vi "set origin.vi"(8 "error in (no error)":errorcluster, 11 "StageMG100204SutterMP285 in":refnum<class "StageMG100204SutterMP285.lvclass">=refnum) -> (0 "error out":errorcluster, 3 "StageMG100204SutterMP285 out":refnum<class "StageMG100204SutterMP285.lvclass">)   [LabVIEW 2010, in "StageMG100204SutterMP285.lvclass"]
uses:
  StageMG100204SutterMP285.lvclass
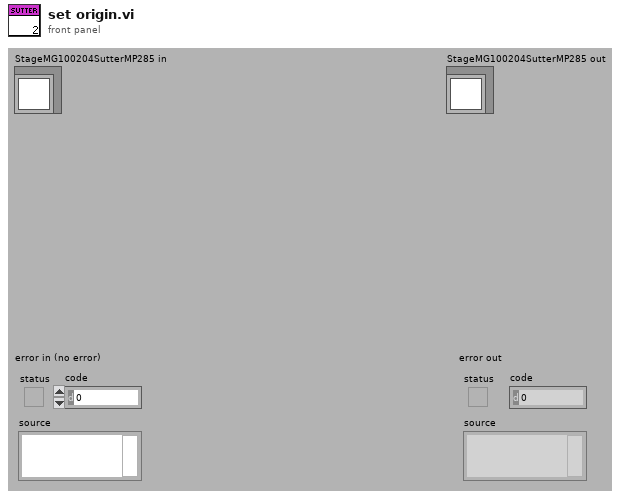
[diagram p1: front panel]
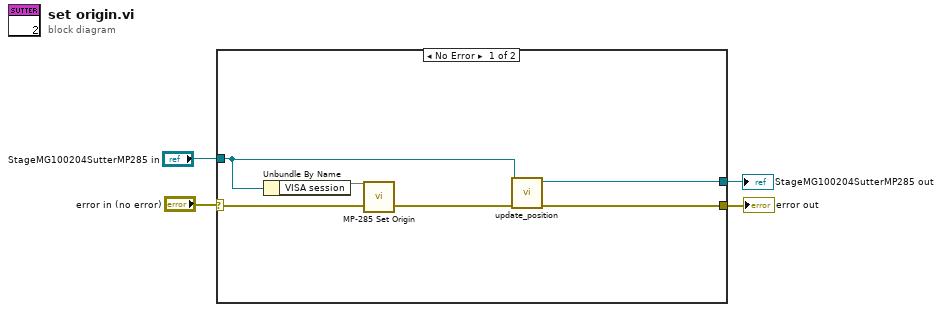
[diagram p0: block diagram]
diagram:
  n1 = case shown="No Error" "error in (no error)" {
    selector: "error in (no error)" -> [w9 w12]
    tunnel: [w7 w12] -> w3
    tunnel: [w5 w11] -> w2
    tunnel: "StageMG100204SutterMP285 in" -> [w6 w11]
    frame No Error {
      n2 = Unbundle By Name(w6) -> ("VISA session"=w10)
      n3 = call "MP-285 Set Origin.vi"("error in (no error)"=w9, "VISA resource name"=w10) -> ("error out"=w8:errorcluster)  [unwired: 1 out]
      n4 = call-dynamic "update_position.vi"("error in (no error)"=w8, "StageMG100204SutterMP285 in"=w6) -> ("error out"=w7:errorcluster, "StageMG100204SutterMP285 out"=w5:refnum<class "StageMG100204SutterMP285.lvclass">)  [unwired: 8 in]
    }
    frame Error {
    }
  }
  "error out" <- w3
  "StageMG100204SutterMP285 out" <- w2
